vi "Get Pin Map ID for Sequence.vi"(8 "error in":errorcluster, 11 "sequence context in":refnum<k7>) -> (0 "error out":errorcluster, 2 "pin map id":string, 3 "sequence context out":refnum<k7>)   [LabVIEW 2020, in "Measurement Plugin TestStand Integration.lvlib"]
doc: "Gets the pin map ID for a TestStand sequence."
uses:
  Measurement Plugin TestStand Integration.lvlib
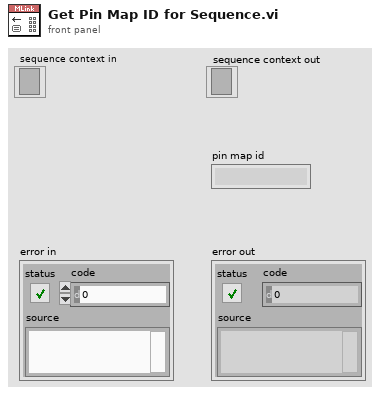
[diagram p1: front panel]
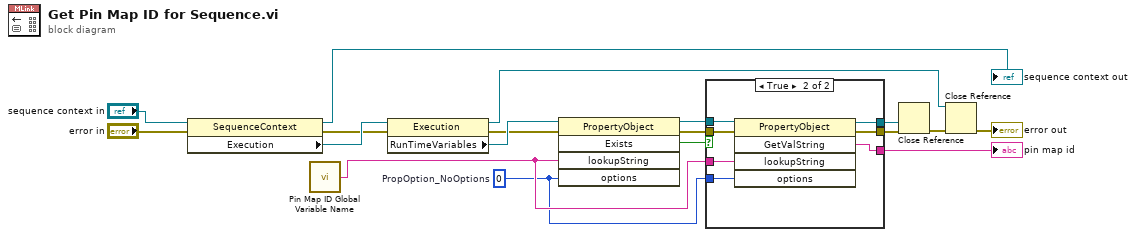
[diagram p0: block diagram]
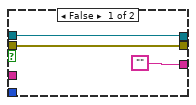
[diagram p2: hidden frame]
diagram:
  w4 = 0  # PropOption_NoOptions
  n1 = property class="SequenceContext"(reference="sequence context in", error in="error in") -> (reference out=→"sequence context out":refnum<k7>, error out=w16:errorcluster, "Execution"=w17:refnum<k7>)
  n2 = call "Pin Map ID Global Variable Name.vi"() -> ("global variable name"=w5:string)
  n3 = property class="Execution"(reference=w17, error in=w16) -> (reference out=w18:refnum<k7>, error out=w9:errorcluster, "RunTimeVariables"=w10:refnum<k7>)
  n4 = invoke class="PropertyObject" method="Exists"(reference=w10, error in=w9, "lookupString"=w5, "options"=w4) -> (reference out=w7:refnum<k7>, error out=w6:errorcluster, "Exists"=w8:bool)  [unwired: 1 in, 2 out]
  n5 = case shown="True" w8 {
    tunnel: [w21 w22] -> w1
    tunnel: ["" w28] -> w12
    tunnel: w7 -> [w19 w27]
    tunnel: w6 -> [w21 w26]
    tunnel: w5 -> [_ w25]
    tunnel: w4 -> [_ w24]
    tunnel: [w19 w23] -> w3
    frame False {
    }
    frame True {
      n6 = invoke class="PropertyObject" method="GetValString"(reference=w27, error in=w26, "lookupString"=w25, "options"=w24) -> (reference out=w23:refnum<k7>, error out=w22:errorcluster, "GetValString"=w28:string)  [unwired: 1 in, 2 out]
    }
  }
  "pin map id" <- w12
  n7 = Close Reference(reference=w3, error in (no error)=w1) -> (error out=w2:errorcluster)
  n8 = Close Reference(reference=w18, error in (no error)=w2) -> (error out=→"error out":errorcluster)
